vi "ConfigureTags.vi"(7 "Sensor Groups (false)":bool, 8 "error in (no error)":errorcluster, 11 "config in":T3) -> (0 "error out":errorcluster, 1 "Registrations":T1[](array[typedef]), 2 "Start OPC Client":bool=TRUE, 3 "config out":T3)   [LabVIEW 2017, in "OPCUAClient.lvlib"]
uses:
  <vilib>/addons/InsightCM/Devices/Shared/Common/OPCUAClient/OPCUAClient.lvlib
  <vilib>/addons/InsightCM/Devices/Shared/Common/OPCUAClient/controls/config.ctl
  <vilib>/OPCUA/controls/OPC UA Client Refnum.ctl
  <vilib>/addons/InsightCM/Devices/Shared/Common/OPCUAClient/controls/group.ctl
  <vilib>/addons/InsightCM/Devices/Shared/Common/OPCUAClient/controls/tag.ctl
  <vilib>/addons/InsightCM/Devices/Shared/Common/DataEventCreator/controls/RegisterTrendPoints.ctl
  <vilib>/addons/InsightCM/Devices/Shared/Common/DataEventCreator/controls/Registry_Trend.ctl
  <vilib>/addons/InsightCM/MessageBus/Base/controls/R2_Channel.ctl
  <vilib>/addons/InsightCM/MessageBus/Base/controls/KeyValuePair.ctl
  <vilib>/addons/InsightCM/MessageBus/Base/controls/Metric.ctl
  <vilib>/addons/PointValueMap/subVIs/Point_Create_double.vi
  <vilib>/addons/InsightCM/Utilities/GlobalConfiguration/GlobalConfiguration.lvlib
  <vilib>/addons/InsightCM/Utilities/PropertyHelpers/PropertyHelpers.lvlib
  <vilib>/addons/InsightCM/Devices/Shared/Common/DataEventCreator/DataEventCreator.lvlib
  <vilib>/addons/PointValueMap/PointValueMap.lvlib
  <vilib>/addons/InsightCM/Utilities/DeviceModelHelpers/DeviceModelHelpers.lvlib
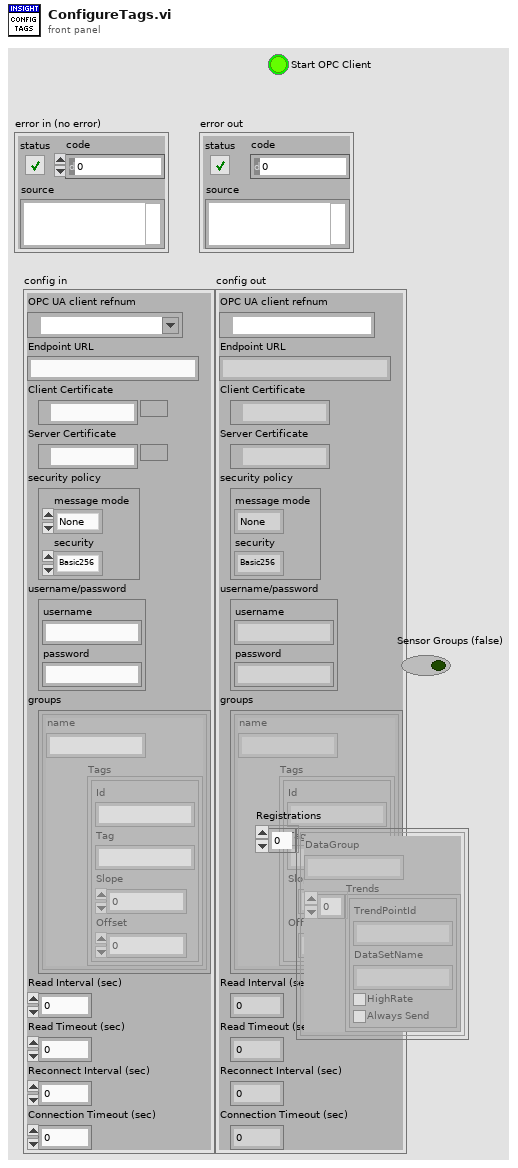
[diagram p1: front panel]
types:
  T1 = typedef "DataEventCreator.lvlib/RegisterTrendPoints.ctl" = cluster{"DataGroup":string, "Trends":T2[]}
  T2 = typedef "DataEventCreator.lvlib/Registry_Trend.ctl" = cluster{"TrendPointId":string, "DataSetName":string, "HighRate":bool, "Always Send":bool}
  T3 = typedef "OPCUAClient.lvlib/config.ctl" = cluster{"OPC UA client refnum":T4, "Endpoint URL":string, "Client Certificate":path, "Server Certificate":path, "security policy":cluster{"message mode":enum16{"None", "Sign", "Sign and Encrypt"}, "security":enum16{"Basic256", "Basic128Rsa15"}}, "username/password":cluster{"username":string, "password":string}, "groups":T5[], "Read Interval (sec)":dbl, "Read Timeout (sec)":dbl, "Reconnect Interval (sec)":dbl, "Connection Timeout (sec)":dbl}
  T4 = typedef "OPC UA Client Refnum.ctl" = refnum<k21>
  T5 = typedef "OPCUAClient.lvlib/group.ctl" = cluster{"name":string, "Tags":T6[]}
  T6 = typedef "OPCUAClient.lvlib/tag.ctl" = cluster{"Id":string, "Tag":string, "Slope":dbl, "Offset":dbl}
  T7 = typedef "AssetNode.ctl" = cluster{"Id":string, "Type":string, "Name":string, "ParentIds":string[], "State":T8, "MeasType":string, "Properties":T9[], "SensorGroups":T10[], "OperatingStates":T13[], "Metrics":T15[], "TrendAlarmRules":T16[], "References":T19[]}
  T8 = typedef "AssetState.ctl" = cluster{"Disabled":bool}
  T9 = typedef "KeyValuePair.ctl" = cluster{"Key":string, "Value":string}
  T10 = typedef "AssetNodeSensorGroup.ctl" = cluster{"Id":string, "Type":string, "SensorIds":string[], "CollectionConfig":T11, "Properties":T9[]}
  T11 = typedef "WirelessCollectionConfig.ctl" = cluster{"GateCondition":T12, "CronString":string, "RetryIntervalMinutes":string, "MaxRetryAttempts":string}
  T12 = typedef "Condition.ctl" = cluster{"Source":string, "Type":string, "Operator":string, "CompareTo":string, "DwellSeconds":dbl}
  T13 = typedef "OperatingState.ctl" = cluster{"Name":string, "Properties":T9[], "Triggers":T14[]}
  T14 = typedef "Trigger.ctl" = cluster{"Type":string, "Expression":string, "Conditions":T12[]}
  T15 = typedef "Metric.ctl" = cluster{"Id":string, "Name":string, "Unit":string, "Properties":T9[], "MetricDefinitionInstanceId":string}
  T16 = typedef "TrendAlarmRule.ctl" = cluster{"Id":string, "AssetNodeId":string, "TrendId":string, "Disabled":bool, "OperatingState":string, "Operator":string, "Hysteresis":dbl, "OnDelaySeconds":dbl, "OffDelaySeconds":dbl, "Levels":T17[], "Properties":T9[]}
  T17 = typedef "TrendAlarmLevel.ctl" = cluster{"Severity":i32, "CompareTo":dbl, "Actions":T18[]}
  T18 = typedef "AlarmAction.ctl" = cluster{"Type":string, "Props":T9[]}
  T19 = typedef "AssetNodeReference.ctl" = cluster{"NodeId":string, "Name":string}
  T20 = typedef "R2_Channel.ctl" = cluster{"Id":string, "DeviceId":string, "Name":string, "ChannelType":string, "HardwareKey":string, "HardwareChannel":string, "DataGroup":string, "Keywords":string[], "EquipmentIds":string[], "Properties":T9[], "Metrics":T15[], "AssetNodeId":string, "MeasType":string, "AssetName":string}
  T21 = typedef "R2_Device.ctl" = cluster{"Id":string, "Name":string, "DeviceType":string, "HardwareName":string, "IpAddress":string, "HardwareInfo":T9[], "ApplicationType":string, "ApplicationVersion":string, "EquipmentIds":string[], "ConfigurationVersion":string, "State":T22, "Properties":T9[], "DataGroups":T23[], "BurstModeTrigger":T24, "SensorGroups":T25[], "Endpoints":T26[]}
  T22 = typedef "DeviceState.ctl" = cluster{"Disabled":bool}
  T23 = typedef "R2_DataGroup.ctl" = cluster{"Name":string, "OperatingStates":T13[], "Properties":T9[], "EquipmentIds":string[], "AssetNodeId":string}
  T24 = typedef "BurstModeTrigger.ctl" = cluster{"Trigger":T14, "SampleRate":string, "AcquisitionLength":string}
  T25 = typedef "DeviceSensorGroup.ctl" = cluster{"EquipId":string, "SensorGroupId":string}
  T26 = typedef "WirelessEndpoint.ctl" = cluster{"SerialNumber":string, "Properties":T9[], "Channels":T27[]}
  T27 = typedef "WirelessChannel.ctl" = cluster{"ChannelNumber":i32, "AssetId":string}
  T28 = typedef "DataSource.ctl" = cluster{"Id":string, "Type":string, "Name":string, "MeasType":string, "Properties":T9[]}
  T29 = typedef "PointValueMap.lvlib/PointMap.ctl" = refnum<data-value>
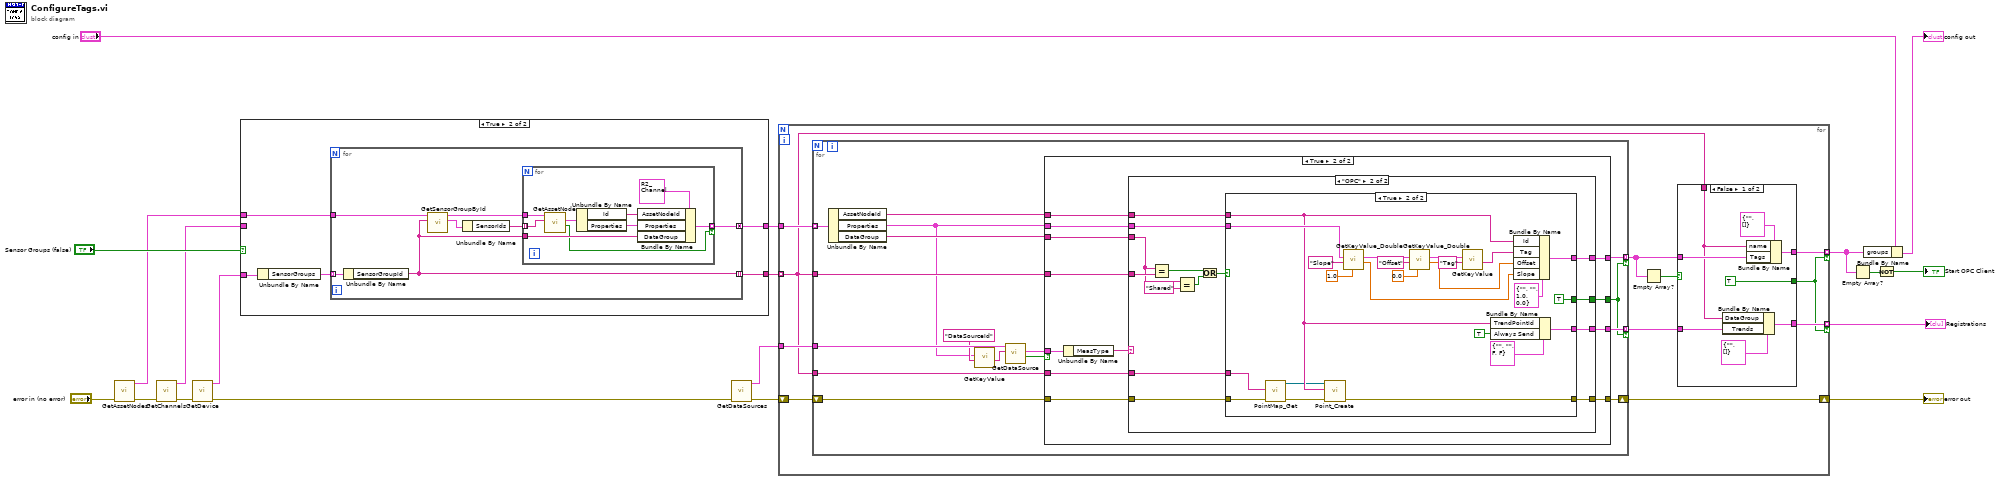
[diagram p0: block diagram]
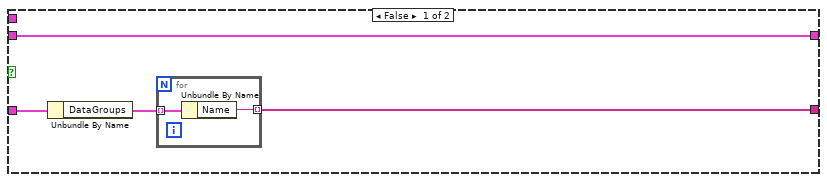
[diagram p2: hidden frame]
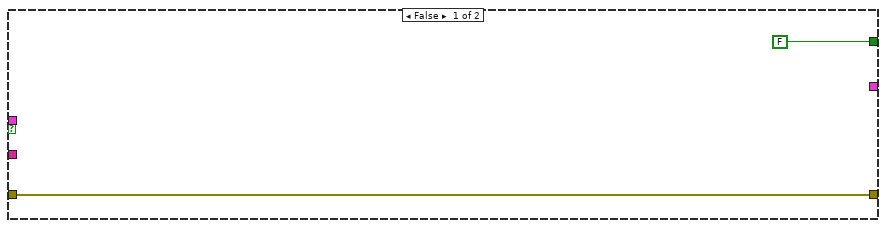
[diagram p3: hidden frame]
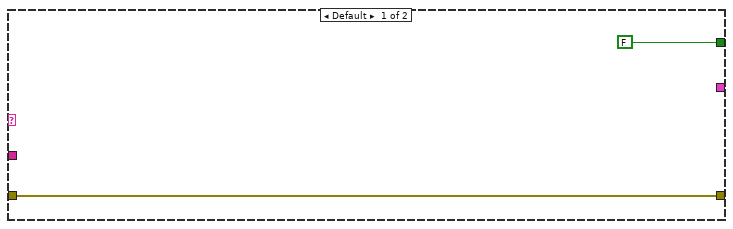
[diagram p4: hidden frame]
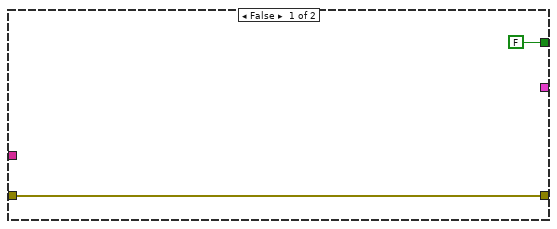
[diagram p5: hidden frame]
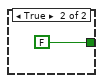
[diagram p6: hidden frame]
diagram:
  n1 = call <vilib>:"GetAssetNodes.vi"("error in (no error)"="error in (no error)") -> ("error out"=w6:errorcluster, "AssetNodes"=w1:T7[])  [unwired: 8 in, 1 out]
  n2 = call <vilib>:"GetChannels.vi"("error in (no error)"=w6) -> ("error out"=w18:errorcluster, "channels"=w2:T20[])  [unwired: 8 in, 1 out]
  n3 = call <vilib>:"GetDevice.vi"("error in (no error)"=w18) -> ("error out"=w10:errorcluster, "device configuration"=w19:T21)  [unwired: 8 in, 1 out]
  n4 = case shown="True" "Sensor Groups (false)" {
    tunnel: w19 -> [w23 w30]
    tunnel: [w21 w28] -> w4
    tunnel: [w20 w26] -> w3
    tunnel: w2 -> [w20 _]
    tunnel: w1 -> [_ w27]
    frame False {
      n5 = Unbundle By Name(w23) -> ("DataGroups"=w22:T23[])
      n6 = for {
        tunnel: w22 -> [w25] mode=indexing
        tunnel: [w24] -> w21 mode=indexing
        n7 = Unbundle By Name(w25) -> ("Name"=w24:string)
      }
    }
    frame True {
      n8 = Unbundle By Name(w30) -> ("SensorGroups"=w29:T25[])
      n9 = for {
        tunnel: w29 -> [w37] mode=indexing
        tunnel: [w32] -> w28 mode=indexing
        tunnel: w27 -> [w36]
        tunnel: [w31] -> w26 mode=concatenating
        n10 = Unbundle By Name(w37) -> ("SensorGroupId"=w32:string)
        n11 = call <vilib>:"GetSensorGroupById.vi"("sensor group id"=w32, "asset nodes in"=w36) -> ("sensor group"=w35:T10, "asset nodes out"=w34:T7[])  [unwired: 7 in, 1 out]
        n12 = Unbundle By Name(w35) -> ("SensorIds"=w33:string[])
        n13 = for {
          tunnel: w34 -> [w45]
          tunnel: w33 -> [w44] mode=indexing
          tunnel: w32 -> [w40]
          tunnel: [w39] -> w31 mode=indexing if=w38
          n14 = call <vilib>:"GetAssetNode.vi"("node id"=w44, "nodes in"=w45) -> ("found"=w38:bool, "AssetNode"=w43:T7)  [unwired: 7 in, 1 out]
          n15 = Unbundle By Name(w43) -> ("Id"=w42:string, "Properties"=w41:T9[])
          n16 = Bundle By Name(cluster=T20 {"Id"="", "DeviceId"="", "Name"="", "ChannelType"="", "HardwareKey"="", "HardwareChannel"="", "DataGroup"="", "Keywords"=[], "EquipmentIds"=[], "Properties"=[], "Metrics"=[], "AssetNodeId"="", "MeasType"="", "AssetName"=""} ("ChannelModel"), "AssetNodeId"=w42, "Properties"=w41, "DataGroup"=w40) -> (w39:T20)
        }
      }
    }
  }
  n17 = call <vilib>:"GetDataSources.vi"("error in (no error)"=w10) -> ("error out"=w9:errorcluster, "data sources"=w8:T28[])  [unwired: 8 in, 1 out]
  n18 = for {
    tunnel: w3 -> [w57]
    tunnel: [w55] -> w17 mode=indexing if=w51
    tunnel: [w52] -> w12 mode=indexing if=w51
    shift-right: [w50] -> w11
    shift-left: w9 -> [w48]
    tunnel: w8 -> [w49]
    tunnel: w4 -> [w47] mode=indexing
    n19 = for {
      tunnel: w57 -> [w73] mode=indexing
      tunnel: w47 -> [w72]
      tunnel: [w71] -> w54 mode=indexing if=w65
      tunnel: [w69] -> w53 mode=indexing if=w65
      shift-right: [w67] -> w50
      shift-left: w48 -> [w68]
      tunnel: w49 -> [w64]
      tunnel: w47 -> [w58]
      n20 = Unbundle By Name(w73) -> ("AssetNodeId"=w66:string, "Properties"=w62:T9[], "DataGroup"=w70:string)
      n21 = call <vilib>:"GetKeyValue.vi"("key"="DataSourceId", "key value pairs"=w62) -> ("value"=w61:string)  [unwired: 7 in, 2 out]
      n22 = call <vilib>:"GetDataSource.vi"("data source id"=w61, "data sources in"=w64) -> ("found"=w60:bool, "DataSource"=w59:T28)  [unwired: 7 in, 1 out]
      n23 = case shown="True" w60 {
        tunnel: w72 -> [_ w87]
        tunnel: [_ w86] -> w71
        tunnel: w70 -> [_ w85]
        tunnel: [_ w84] -> w69
        tunnel: w68 -> [w74 w83]
        tunnel: [w74 w82] -> w67
        tunnel: w66 -> [_ w81]
        tunnel: [FALSE ("Always Send") w80] -> w65
        tunnel: w62 -> [_ w79]
        tunnel: w59 -> [_ w78]
        tunnel: w58 -> [_ w76]
        frame False {
        }
        frame True {
          n24 = Unbundle By Name(w78) -> ("MeasType"=w77:string)
          n25 = case shown="\"OPC\"" w77 {
            tunnel: w87 -> [_ w103]
            tunnel: [_ w102] -> w86
            tunnel: w79 -> [_ w101]
            tunnel: w85 -> [_ w92]
            tunnel: [_ w100] -> w84
            tunnel: w83 -> [w89 w99]
            tunnel: [w89 w98] -> w82
            tunnel: w81 -> [_ w97]
            tunnel: [FALSE ("Always Send") w96] -> w80
            tunnel: w76 -> [_ w90]
            frame Default {
            }
            frame "OPC" {
              n26 = Equal?(x=w92, y=w103) -> (x = y?=w95:bool)
              n27 = Equal?(x=w92, y="Shared") -> (x = y?=w93:bool)
              n28 = Or(x=w95, y=w93) -> (x .or. y?=w94:bool)
              n29 = case shown="True" w94 {
                tunnel: [_ w121] -> w102
                tunnel: w101 -> [_ w120]
                tunnel: [_ w115] -> w100
                tunnel: w99 -> [w104 w109]
                tunnel: [w104 w113] -> w98
                tunnel: w97 -> [_ w111]
                tunnel: [FALSE ("Always Send") TRUE ("Always Send")] -> w96
                tunnel: w90 -> [_ w106]
                frame False {
                }
                frame True {
                  n30 = call <vilib>:"PointMap_Get.vi"("error in (no error)"=w109, "Name"=w106) -> ("error out"=w108:errorcluster, "Map Out"=w107:T29)  [unwired: 7 in, 1 out]
                  n31 = call-poly <vilib>:"Point_Create.vi"("Error In"=w108, "Tag"=w111, "Map"=w107) -> ("Error Out"=w113:errorcluster)  [unwired: 7 in, 1 out]
                  n32 = call <vilib>:"GetKeyValue_Double.vi"("default"=1.0, "key"="Slope", "key value pairs"=w120) -> ("value"=w122:dbl, "key value pairs out"=w128:T9[])  [unwired: 6 in, 1 out]
                  n33 = call <vilib>:"GetKeyValue_Double.vi"("default"=0.0, "key"="Offset", "key value pairs"=w128) -> ("value"=w119:dbl, "key value pairs out"=w118:T9[])  [unwired: 6 in, 1 out]
                  n34 = call <vilib>:"GetKeyValue.vi"("key"="Tag", "key value pairs"=w118) -> ("value"=w112:string)  [unwired: 7 in, 2 out]
                  n35 = Bundle By Name(cluster=T2 {"TrendPointId"="", "DataSetName"="", "HighRate"=FALSE, "Always Send"=FALSE} ("Trend"), "TrendPointId"=w111, "Always Send"=TRUE) -> (w115:T2)
                  n36 = Bundle By Name(cluster=T6 {"Id"="", "Tag"="", "Slope"=1.0, "Offset"=0.0} ("OPCUA Tag"), "Id"=w111, "Tag"=w112, "Offset"=w119, "Slope"=w122) -> (w121:T6)
                }
              }
            }
          }
        }
      }
    }
    n37 = Empty Array?(array=w54) -> (empty?=w56:bool)
    n38 = case shown="False" w56 {
      tunnel: [w135 _] -> w55
      tunnel: [TRUE FALSE] -> w51
      tunnel: w54 -> [w133 _]
      tunnel: w53 -> [w131 _]
      tunnel: [w130 _] -> w52
      tunnel: w47 -> [w129 _]
      frame False {
        n39 = Bundle By Name(cluster=T1 {"DataGroup"="", "Trends"=[]} ("register trend"), "DataGroup"=w129, "Trends"=w131) -> (w130:T1)
        n40 = Bundle By Name(cluster=T5 {"name"="", "Tags"=[]} ("group"), "name"=w129, "Tags"=w133) -> (w135:T5)
      }
      frame True {
      }
    }
  }
  "error out" <- w11
  "Registrations" <- w12
  n41 = Empty Array?(array=w17) -> (empty?=w14:bool)
  n42 = Bundle By Name(cluster="config in", "groups"=w17) -> (→"config out":T3)
  n43 = Not(x=w14) -> (.not. x?=→"Start OPC Client":bool)
